vi "Open NART Connection.vi"(0 "NART Directory":path, 5 "IP Address (\"\": localhost)":string, 7 "port (2390)":u32=2390, 11 "error in (no error)":errorcluster, 12 "Timeout (2500ms)":i32=2500) -> (4 "NART TCP Connection":refnum<k5>, 15 "error out":errorcluster)   [LabVIEW 2011, in "ART2 Test Panel.lvlib"]
uses:
  ART2 Test Panel.lvlib
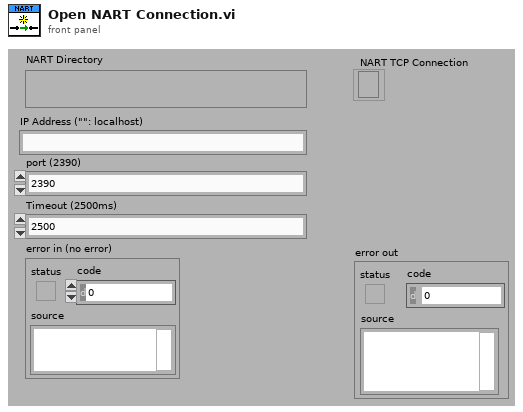
[diagram p1: front panel]
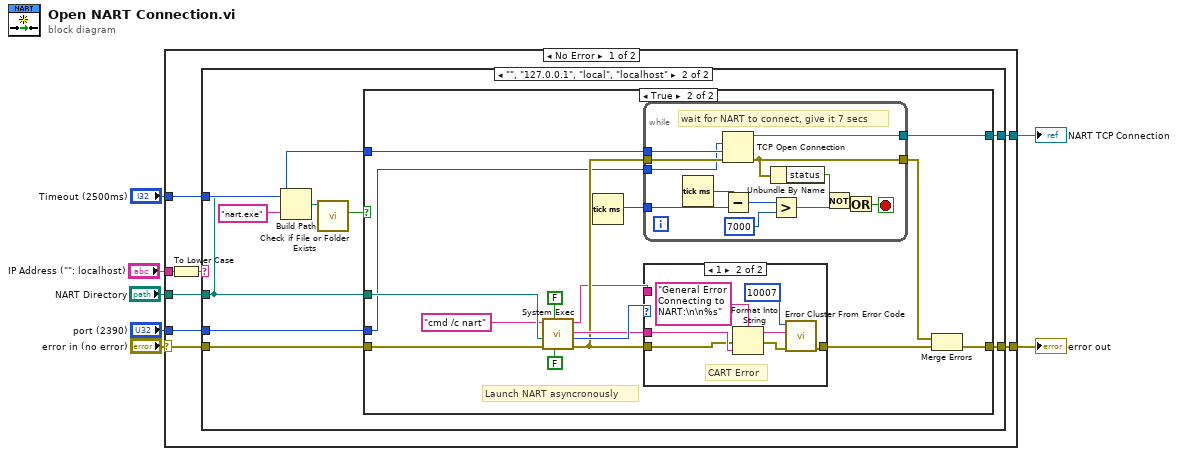
[diagram p0: block diagram]
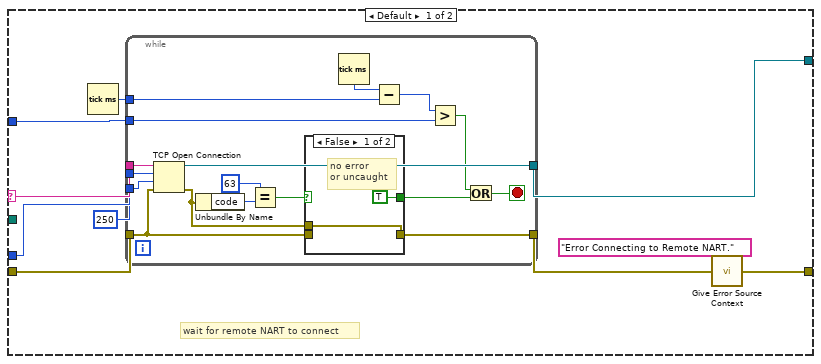
[diagram p2: hidden frame]
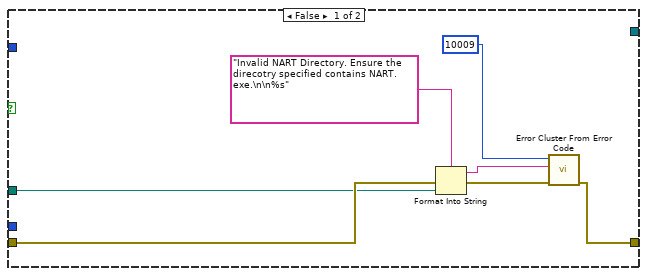
[diagram p4: hidden frame]
diagram:
  n1 = case shown="No Error" "error in (no error)" {
    selector: "error in (no error)" -> [w11 w99]
    tunnel: [w15 w99] -> w3
    tunnel: "Timeout (2500ms)" -> [w14 _]
    tunnel: [w13 _] -> w2
    tunnel: "port (2390)" -> [w12 _]
    tunnel: "NART Directory" -> [w10 _]
    tunnel: "IP Address (\"\": localhost)" -> [w9 _]
    frame No Error {
      n2 = To Lower Case(string=w9) -> (all lower case string=w8:string)
      n3 = case shown="\"\", \"127.0.0.1\", \"local\", \"localhost\"" w8 {
        selector: w8 -> [w25 _]
        tunnel: [w20 w54] -> w15
        tunnel: w14 -> [w17 w53]
        tunnel: [w23 w52] -> w13
        tunnel: w12 -> [w24 w51]
        tunnel: w11 -> [w22 w50]
        tunnel: w10 -> [_ w47]
        frame Default {
          # "wait for remote NART to connect"
          n4 = Tick Count (ms)() -> (millisecond timer value=w18:u32)
          n5 = while {
            tunnel: w25 -> [w42]
            tunnel: w24 -> [w41]
            tunnel: [w40] -> w23
            tunnel: w22 -> [w35]
            tunnel: [w37] -> w21
            tunnel: w18 -> [w32]
            tunnel: w17 -> [w30]
            tunnel: 250 ("timeout ms (60000)") -> [w26]
            stop <- w27 stop-if-true
            n6 = TCP Open Connection(address=w42, remote port or service name=w41, timeout ms (60000)=w26, error in (no error)=w35) -> (connection ID=w40:refnum<k5>, error out=w36:errorcluster)  [unwired: 1 in]
            n7 = Unbundle By Name(w36) -> ("code"=w39:i32)
            n8 = Equal?(x=63, y=w39) -> (x = y?=w34:bool)
            n9 = case shown="False" w34 {
              tunnel: [w44 w45] -> w37
              tunnel: w36 -> [w44 _]
              tunnel: [TRUE ("status") _] -> w28
              tunnel: w35 -> [_ w45]
              frame False {
                # "no error\nor uncaught"
              }
              frame True {
              }
            }
            n10 = Tick Count (ms)() -> (millisecond timer value=w33:u32)
            n11 = Subtract(x=w33, y=w32) -> (x-y=w31:u32)
            n12 = Greater?(x=w31, y=w30) -> (0:w29:bool)
            n13 = Or(x=w29, y=w28) -> (x .or. y?=w27:bool)
          }
          n14 = call "Give Error Source Context.vi"("Context String"="Error Connecting to Remote NART." ("string"), "error in"=w21) -> ("Error out with context"=w20:errorcluster)  [unwired: 13 in]
        }
        frame "", "127.0.0.1", "local", "localhost" {
          n15 = Build Path(base path=w47, name or relative path="nart.exe") -> (appended path=w48:path)
          n16 = call <vilib>:"Check if File or Folder Exists.vi"("path"=w48) -> ("file or folder exists?"=w46:bool)  [unwired: 8 in, 2 out]
          n17 = case shown="True" w46 {
            tunnel: [w57 w77] -> w54
            tunnel: w53 -> [_ w76]
            tunnel: [_ w75] -> w52
            tunnel: w51 -> [_ w66]
            tunnel: w50 -> [w56 w63]
            tunnel: w47 -> [w55 w68]
            frame False {
              n18 = Format Into String(format string="Invalid NART Directory. Ensure the direcotry specified contains NART.exe.\n\n%s", error in=w56, w55) -> (resulting string=w60:string, error out=w58:errorcluster)  [unwired: 1 in]
              n19 = call <vilib>:"Error Cluster From Error Code.vi"("error in (no error)"=w58, "error message (\"\")"=w60, "error code (0)"=10009) -> ("error out"=w57:errorcluster)  [unwired: 6 in]
            }
            frame True {
              # "Launch NART asyncronously"
              n20 = call <vilib>:"System Exec.vi"("run minimized? (F)"=FALSE, "wait until completion? (T)"=FALSE, "error in (no error)"=w63, "working directory"=w68, "command line"="cmd /c nart" ("format string")) -> ("error out"=w67:errorcluster, "return code"=w73:i32, "standard error"=w71:string, "standard output"=w65:string)  [unwired: 3 in]
              n21 = Tick Count (ms)() -> (millisecond timer value=w62:u32)
              n22 = while {
                tunnel: w76 -> [w90]
                tunnel: [w89] -> w75
                tunnel: [w82] -> w74
                tunnel: w67 -> [w88]
                tunnel: w66 -> [w87]
                tunnel: w62 -> [w85]
                stop <- w81 stop-if-true
                # "wait for NART to connect, give it 7 secs"
                n23 = Tick Count (ms)() -> (millisecond timer value=w86:u32)
                n24 = TCP Open Connection(remote port or service name=w87, timeout ms (60000)=w90, error in (no error)=w88) -> (connection ID=w89:refnum<k5>, error out=w82:errorcluster)  [unwired: 2 in]
                n25 = Subtract(x=w86, y=w85) -> (x-y=w84:u32)
                n26 = Unbundle By Name(w82) -> ("status"=w79:bool)
                n27 = Greater?(x=w84, y=u32 7000) -> (0:w80:bool)
                n28 = Not(x=w79) -> (.not. x?=w78:bool)
                n29 = Or(x=w78, y=w80) -> (x .or. y?=w81:bool)
              }
              n30 = case shown="1" w73 {
                tunnel: w67 -> [w91 w93]
                tunnel: [w91 w98] -> w72
                tunnel: w71 -> [_ w94]
                tunnel: w65 -> [_ _]
                frame Default {
                }
                frame 1 {
                  # "CART Error"
                  n31 = Format Into String(format string="General Error Connecting to NART:\n\n%s", error in=w93, w94) -> (resulting string=w96:string, error out=w92:errorcluster)  [unwired: 1 in]
                  n32 = call <vilib>:"Error Cluster From Error Code.vi"("error in (no error)"=w92, "error message (\"\")"=w96, "error code (0)"=10007) -> ("error out"=w98:errorcluster)  [unwired: 6 in]
                }
              }
              n33 = Merge Errors(w74, w72) -> (w77:errorcluster)
            }
          }
        }
      }
    }
    frame Error {
    }
  }
  "error out" <- w3
  "NART TCP Connection" <- w2
